vi "CSM - Compact Multiple States.vi"(9 "Multiple States":string[](array[string])) -> (2 "States":string)   [LabVIEW 2020, in "Communicable State Machine.lvlib"]
doc: "Compact multiple states to a single string for input.\n\n<b>Inputs:</b>\n - <b>States in Lines</b>: Multiple states as string array.\n\n<b>Outputs:</b>\n - <b>States</b>: State String contains all the input state(s)"
uses:
  Communicable State Machine.lvlib
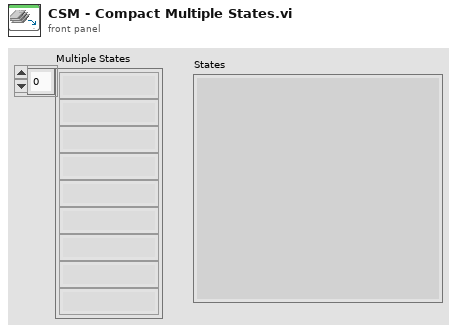
[diagram p1: front panel]
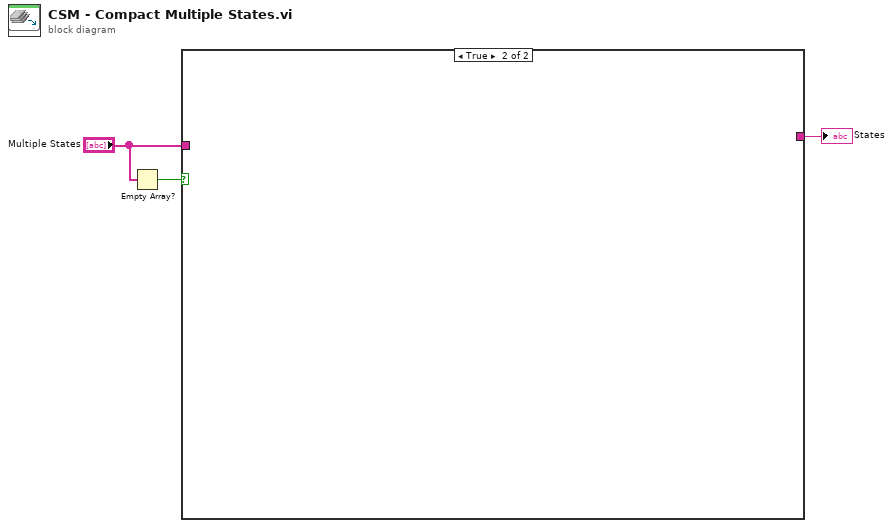
[diagram p0: block diagram]
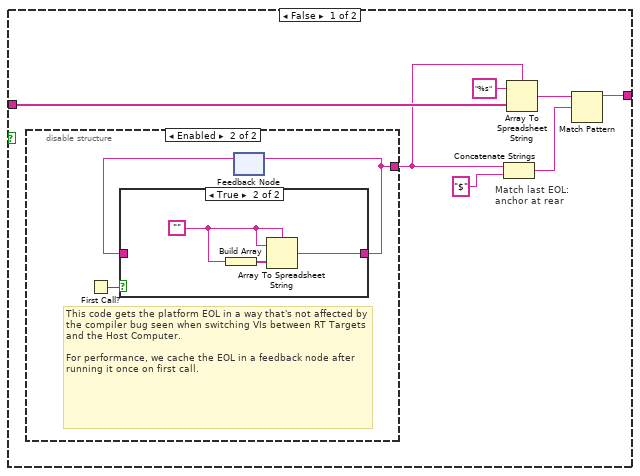
[diagram p2: hidden frame]
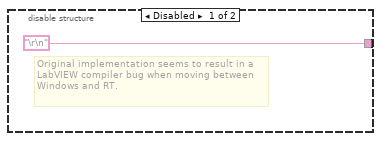
[diagram p3: hidden frame]
diagram:
  n1 = Empty Array?(array="Multiple States") -> (empty?=w1:bool)
  n2 = case shown="True" w1 {
    tunnel: [w10 _] -> w3
    tunnel: "Multiple States" -> [w9 _]
    frame False {
      # "Match last EOL:\nanchor at rear"
      n3 = disable-structure shown="Enabled" {
        disable-tunnel: ["\r\n" w14] -> w4
        frame Disabled {
          # "Original implementation seems to result in a LabVIEW compiler bug when moving between Windows and RT."
        }
        frame Enabled {
          # "This code gets the platform EOL in a way that's not affected by the compiler bug seen when switching VIs between RT Targets and the Host Computer.\n\nFor performance, we cache the EOL in a feedback node after running it once on first call."
          n4 = First Call?() -> (First Call?: T/F=w13:bool)
          n5 = feedback #1() -> (w12:string)  [unwired: 1 in]
          n6 = case shown="True" w13 {
            tunnel: [w15 w16] -> w14
            tunnel: w12 -> [w15 _]
            frame False {
            }
            frame True {
              w17 = "" ("Empty String\n(hidden on FP)")
              n7 = Build Array(w17) -> (w18:string[])
              n8 = Array To Spreadsheet String(delimiter (Tab)=w17, array=w18, 3:w17) -> (spreadsheet string=w16:string)
            }
          }
          n9 = feedback-in #1(w14) -> ()
        }
      }
      n10 = Concatenate Strings(w4, "$" ("Substring")) -> (w7:string)
      n11 = Array To Spreadsheet String(delimiter (Tab)=w4, array=w9, 3:"%s" ("format string")) -> (spreadsheet string=w8:string)
      n12 = Match Pattern(string=w8, regular expression=w7) -> (before substring=w10:string)  [unwired: 1 in, 3 out]
    }
    frame True {
    }
  }
  "States" <- w3
